vi "read.vi"(8 "error in (no error)":errorcluster, 11 "Lakeshore 325 in":refnum<class "Lakeshore 325.lvclass">) -> (0 "error out":errorcluster, 2 "Data":dbl[](array[numeric]), 3 "Lakeshore 325 out":refnum<class "Lakeshore 325.lvclass">)   [LabVIEW 2022 SP3, in "Lakeshore 325.lvclass"]
uses:
  Lakeshore 325.lvclass
  Lakeshore 325.lvclass/Lakeshore 325.ctl
  <instrlib>/Lake Shore 325/Lake Shore 325.lvlib
  <instrlib>/Lake Shore 325/Public/Data/Sensor Data (Single Reading).vi
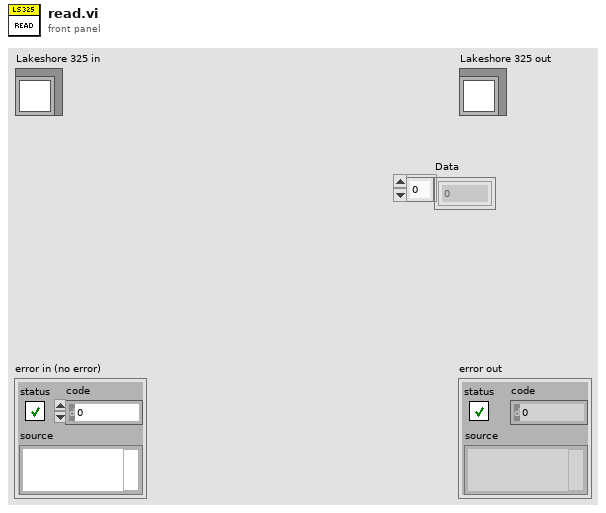
[diagram p1: front panel]
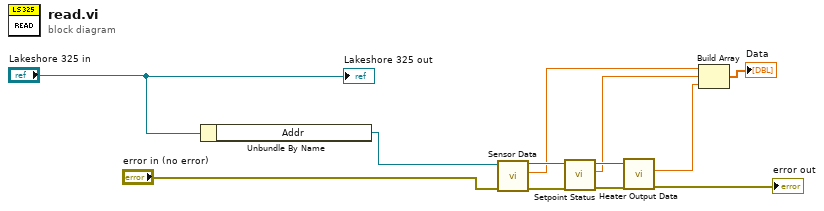
[diagram p0: block diagram]
diagram:
  n1 = Unbundle By Name("Lakeshore 325 in") -> ("Addr"=w12:refnum<visa-resource-name>)
  n2 = call-poly <instrlib>:"Sensor Data.vi"("error in (no error)"="error in (no error)", "VISA resource name"=w12) -> ("error out"=w10:errorcluster, "Sensor Data"=w3:dbl, "VISA resource name out"=w9:refnum<visa-resource-name>)  [unwired: 7 in]
  n3 = call <instrlib>:"Setpoint Status.vi"("error in (no error)"=w10, "VISA resource name"=w9) -> ("error out"=w8:errorcluster, "Setpoint Value"=w4:dbl, "VISA resource name out"=w7:refnum<visa-resource-name>)  [unwired: 7 in]
  n4 = call <instrlib>:"Heater Output Data.vi"("error in (no error)"=w8, "VISA resource name"=w7) -> ("error out"=→"error out":errorcluster, "Heater Output Value"=w5:dbl)  [unwired: 7 in, 1 out]
  n5 = Build Array(w3, w4, w5) -> (→"Data":dbl[])
  "Lakeshore 325 out" <- "Lakeshore 325 in"
